vi "Setpoint.vi"(8 "ZENONE.Q_set [kVAr]":dbl, 9 "ZENONE.P_set [kW]":dbl, 11 "setpoints IN":dbl[](array[numeric])) -> (2 "OUT":T1)   [LabVIEW 2021]
uses:
  Setpoints_CDA.ctl
  Setpoints_CDA_ZENONE.ctl
panel:
  in  "delta_BESS":dbl format="%#_13g"
  # "PV Curtail [%]"
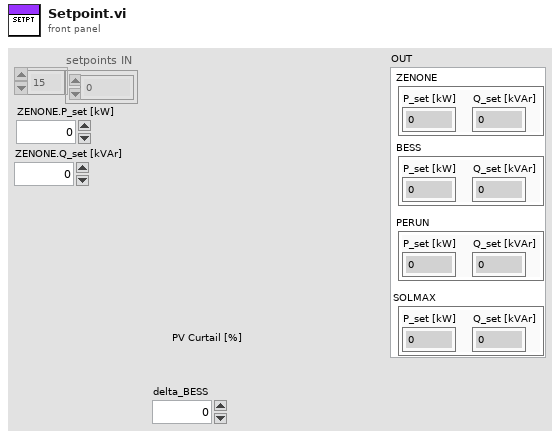
[diagram p1: front panel]
types:
  T1 = typedef "Setpoints_CDA.ctl" = cluster{"ZENONE":T2, "BESS":T2, "PERUN":T2, "SOLMAX":T2}
  T2 = typedef "Setpoints_CDA_ZENONE.ctl" = cluster{"P_set [kW]":dbl, "Q_set [kVAr]":dbl}
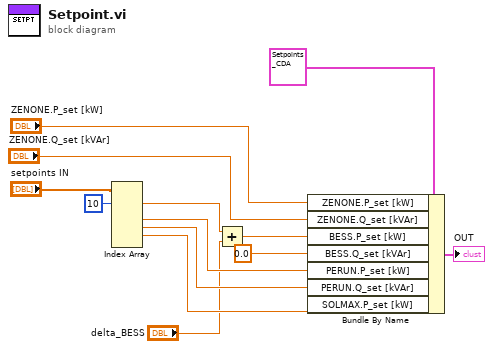
[diagram p0: block diagram]
diagram:
  n1 = Index Array(array="setpoints IN", index #1=10 ("index")) -> (element #1=w10:dbl, element #3=w9:dbl, element #4=w8:dbl, element #5=w3:dbl)  [unwired: 5 in, 2 out]
  n2 = Add(x=w10, y="delta_BESS") -> (x+y=w2:dbl)
  n3 = Bundle By Name(cluster=T1 {"ZENONE"={"P_set [kW]"=0.0, "Q_set [kVAr]"=0.0}, "BESS"={"P_set [kW]"=0.0, "Q_set [kVAr]"=0.0}, "PERUN"={"P_set [kW]"=0.0, "Q_set [kVAr]"=0.0}, "SOLMAX"={"P_set [kW]"=0.0, "Q_set [kVAr]"=0.0}} ("CDA_setpoints"), "ZENONE.P_set [kW]"="ZENONE.P_set [kW]", "ZENONE.Q_set [kVAr]"="ZENONE.Q_set [kVAr]", "BESS.P_set [kW]"=w2, "BESS.Q_set [kVAr]"=0.0 ("BESS.Q_set"), "PERUN.P_set [kW]"=w9, "PERUN.Q_set [kVAr]"=w8, "SOLMAX.P_set [kW]"=w3) -> (→"OUT":T1)
